vi "Close Ref.vi"(8 "error in (no error)":errorcluster, 11 "Listener In.lvclass":refnum<class "Listener.lvclass">) -> (0 "error out":errorcluster)   [LabVIEW 2019, in "Listener.lvclass"]
uses:
  Listener.lvclass
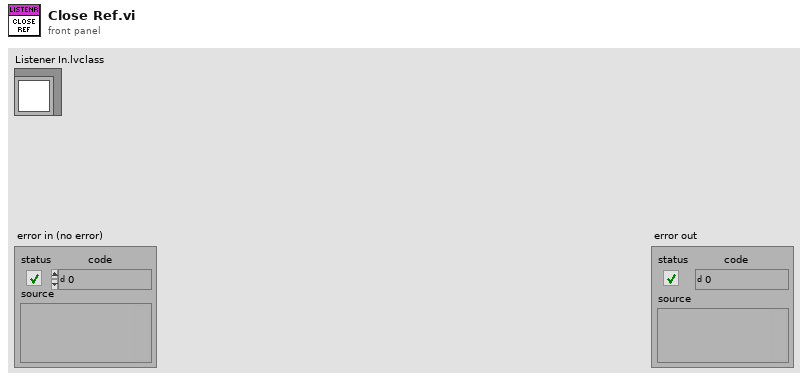
[diagram p1: front panel]
types:
  T1 = typedef "Listener.lvclass/Protocol Ctl.ctl" = enum16{"RS-XXX", "VISA", "TCPIP", "UDP", "GPIB ConvBox"}
  T2 = typedef "Listener.lvclass/TCP IP Data Structure.ctl" = cluster{"TCP|IP connection ID":refnum<k5>, "IP Address":string, "Port":u16, "Data":string}
  T3 = typedef "Listener.lvclass/UDP Data Structure.ctl" = cluster{"UDP connection ID":refnum<k16>, "Local Address":string, "Local Port":u16, "Target IP Address":string, "Target Port":u16, "Data":string}
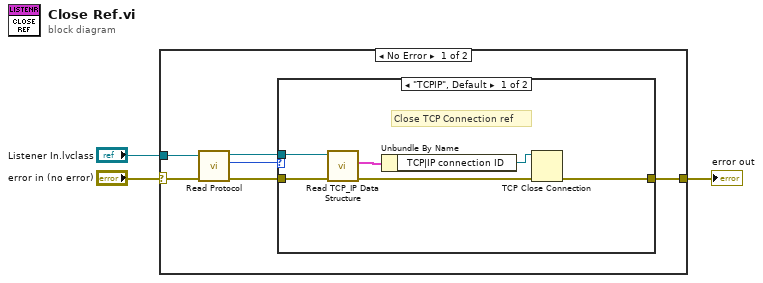
[diagram p0: block diagram]
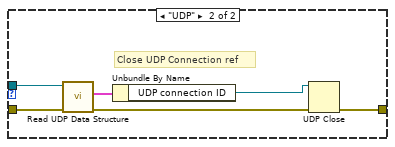
[diagram p2: hidden frame]
diagram:
  n1 = case shown="No Error" "error in (no error)" {
    selector: "error in (no error)" -> [w6 w22]
    tunnel: [w4 w22] -> w2
    tunnel: "Listener In.lvclass" -> [w9 _]
    frame No Error {
      n2 = call-dynamic "Read Protocol.vi"("error in (no error)"=w6, "Listener in"=w9) -> ("error out"=w5:errorcluster, "Protocol"=w8:T1, "Listener out"=w7:refnum<class "Listener.lvclass">)  [unwired: 7 in]
      n3 = case shown="\"TCPIP\", Default" w8 {
        tunnel: w7 -> [w14 w21]
        tunnel: w5 -> [w15 w20]
        tunnel: [w11 w16] -> w4
        frame "TCPIP", Default {
          # "Close TCP Connection ref"
          n4 = call-dynamic "Read TCP_IP Data Structure.vi"("error in (no error)"=w15, "Listener in"=w14) -> ("error out"=w12:errorcluster, "TCP|IP Data Structure"=w13:T2)  [unwired: 7 in, 1 out]
          n5 = Unbundle By Name(w13) -> ("TCP|IP connection ID"=w10:refnum<k5>)
          n6 = TCP Close Connection(connection ID=w10, error in (no error)=w12) -> (error out=w11:errorcluster)  [unwired: 1 in, 1 out]
        }
        frame "UDP" {
          # "Close UDP Connection ref"
          n7 = call-dynamic "Read UDP Data Structure.vi"("error in (no error)"=w20, "Listener in"=w21) -> ("error out"=w18:errorcluster, "UDP Data Structure"=w19:T3)  [unwired: 7 in, 1 out]
          n8 = Unbundle By Name(w19) -> ("UDP connection ID"=w17:refnum<k16>)
          n9 = UDP Close(connection ID=w17, 8:w18) -> (error out=w16:errorcluster)  [unwired: 1 out]
        }
      }
    }
    frame Error {
    }
  }
  "error out" <- w2
